vi "Remove Created.vi"(9 "Self Alias":string, 10 "Addresses DVR in":refnum<data-value>) -> (0 "error out":errorcluster, 2 "Addresses DVR out":refnum<data-value>)   [LabVIEW 2021, in "jettl.lvlib" / "Addresses.lvlib"]
uses:
  Addresses.lvlib
  Addresses/Addresses.lvclass
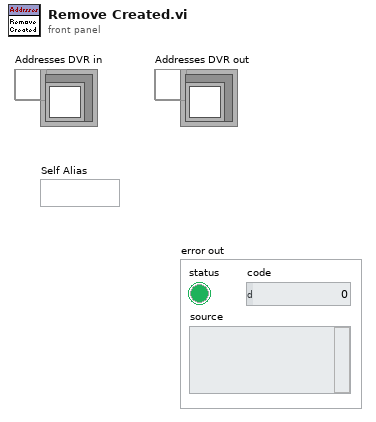
[diagram p1: front panel]
types:
  T1 = typedef "jettl.lvlib/Addresses.lvlib/Created.ctl" = map{string, refnum<class "Msg Type Strategy.lvclass">}
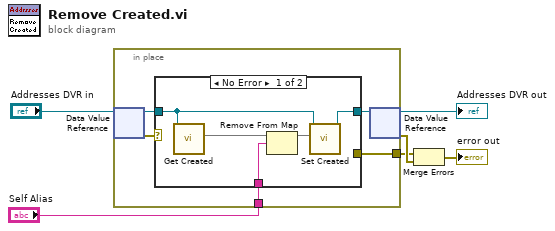
[diagram p0: block diagram]
diagram:
  n1 = in-place {
    in-place-border: [w11] -> w2
    in-place-border: "Self Alias" -> [w8]
    n2 = in-place-dvr #1("Addresses DVR in") -> (w9:refnum<class "Addresses.lvclass">, w10:errorcluster)
    n3 = case shown="No Error" w10 {
      selector: w10 -> [_ w18]
      tunnel: w9 -> [w13 w17]
      tunnel: [_ w18] -> w11
      tunnel: w8 -> [w15 _]
      tunnel: [w12 w17] -> w7
      frame No Error {
        n4 = call "Get Created.vi"("Addresses in"=w13) -> ("Created"=w16:T1)  [unwired: 10 in]
        n5 = Remove From Map(10:w15, 11:w16) -> (3:w14:T1)  [unwired: 2 out]
        n6 = call "Set Created.vi"("Created"=w14, "Addresses in"=w13) -> ("Addresses out"=w12:refnum<class "Addresses.lvclass">)  [unwired: 9 in]
      }
      frame Error {
      }
    }
    n7 = in-place-dvr #1(w7) -> (→"Addresses DVR out":refnum<data-value>, w3:errorcluster)
  }
  n8 = Merge Errors(w2, w3) -> (→"error out":errorcluster)
